vi "set exposure time.vi"(8 "error in (no error)":errorcluster, 11 "Thorcam in":refnum<class "Thorcam.lvclass">) -> (0 "error out":errorcluster, 3 "Thorcam out":refnum<class "Thorcam.lvclass">)   [LabVIEW 2012, in "Thorcam.lvclass"]
uses:
  Thorcam.lvclass
  Thorcam.lvclass/Thorcam.ctl
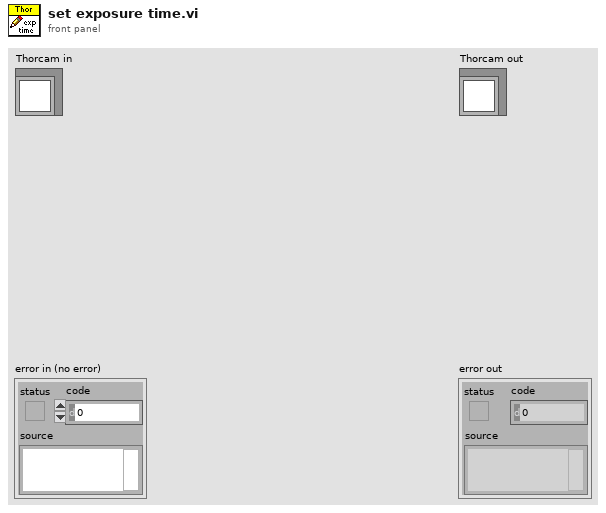
[diagram p1: front panel]
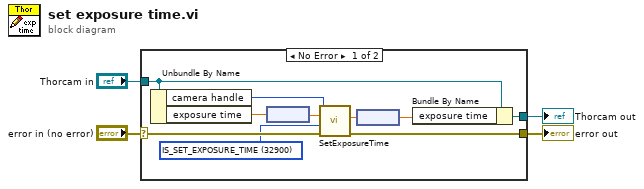
[diagram p0: block diagram]
diagram:
  n1 = case shown="No Error" "error in (no error)" {
    selector: "error in (no error)" -> [w12 w16]
    tunnel: [w11 w16] -> w3
    tunnel: [w5 w15] -> w1
    tunnel: "Thorcam in" -> [w6 w15]
    frame No Error {
      w10 = u16 32900 items=["IS_SET_EXPOSURE_TIME"=32900, "IS_GET_EXPOSURE_TIME"=32768, "IS_GET_DEFAULT_EXPOSURE"=32769] ("Mode")
      n2 = Unbundle By Name(w6) -> ("camera handle"=w14:u32, "exposure time"=w13:dbl[unit])
      n3 = node(w13) -> (w9:dbl)
      n4 = call <instrlib>:"SetExposureTime.vi"("error in"=w12, "Mode"=w10, "Exposure Time"=w9, "Camera Handle In"=w14) -> ("error out"=w11:errorcluster, "new exposure time"=w7:dbl)  [unwired: 5 in, 1 out]
      n5 = node(w7) -> (w8:dbl[unit])
      n6 = Bundle By Name(cluster=w6, "exposure time"=w8) -> (w5:refnum<class "Thorcam.lvclass">)
    }
    frame Error {
    }
  }
  "error out" <- w3
  "Thorcam out" <- w1
